vi "Write.vi"(8 "error in (no error)":errorcluster, 10 "Write":string, 11 "WebSocket in":refnum<class "WebSocket.lvclass">) -> (0 "error out":errorcluster, 3 "WebSocket out":refnum<class "WebSocket.lvclass">)   [LabVIEW 2021, in "WebSocket.lvlib" / "WebSocket.lvclass"]
uses:
  WebSocket.lvclass
  WebSocket.lvclass/WebSocket.ctl
  <vilib>/MediaMongrels Ltd/WebSockets/WebSockets/WebSocket Server/WebSocket Server.lvclass
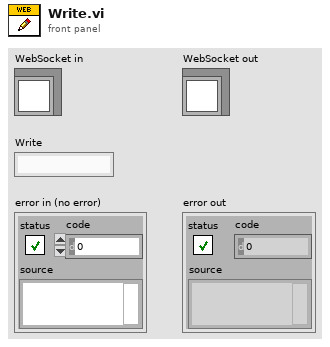
[diagram p1: front panel]
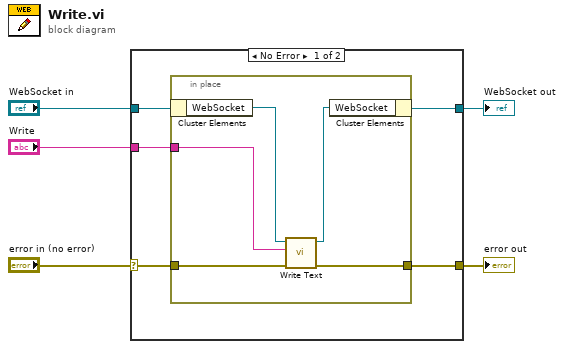
[diagram p0: block diagram]
diagram:
  n1 = case shown="No Error" "error in (no error)" {
    selector: "error in (no error)" -> [w8 w17]
    tunnel: [w7 w17] -> w4
    tunnel: [w6 w16] -> w2
    tunnel: "WebSocket in" -> [w10 w16]
    tunnel: "Write" -> [w9 _]
    frame No Error {
      n2 = in-place {
        in-place-border: w9 -> [w13]
        in-place-border: w8 -> [w12]
        in-place-border: [w11] -> w7
        n3 = in-place-cluster #1(w10) -> ("WebSocket"=w15:refnum<class "WebSocket Server.lvclass">)
        n4 = call-dynamic "Write Text.vi"("error in (no error)"=w12, "String Data"=w13, "WebSocket in"=w15) -> ("error out"=w11:errorcluster, "WebSocket out"=w14:refnum<class "WebSocket Server.lvclass">)  [unwired: 7 in]
        n5 = in-place-cluster #1("WebSocket"=w14) -> (w6:refnum<class "WebSocket.lvclass">)
      }
    }
    frame Error {
    }
  }
  "error out" <- w4
  "WebSocket out" <- w2
